vi "Single Point CW.vi"() -> ()   [LabVIEW 2020]
uses:
  Labview Library/Libraries/Basic Experiment/CW Results.ctl
  Labview Library/Libraries/Basic Experiment/CW Fit Frequency.ctl
  <vilib>/Math Plots/2D Math Plots/2D Error Bar/2D Error Bar XCtrl/2D Error Bar.xctl
  <vilib>/Math Plots/2D Math Plots/2D Error Bar/2D Error Bar Datatype/2D Error Bar Datatype.lvclass
  Labview Library/Libraries/Basic Experiment/CW settings.ctl
  Labview Library/Libraries/Basic Experiment/AutoTrace Setting For Exp.ctl
  Labview Library/Libraries/HW_LMMR_ASG8100/LMMR ASG/ASG Instructions XControl.xctl
  <vilib>/Analysis/baseanly.llb/Mean (DBL).vi
  <vilib>/Math Plots/2D Math Plots/2D Error Bar/2D Error Bar Datatype/Public/Plot Helper (Percentage).vi
  Labview Library/Libraries/Basic Experiment/Basic Experiment.lvlib
  Labview Library/Libraries/UT_Utilities/Utilities.lvlib
  Labview Library/Libraries/HW_LMMR_ASG8100/LMMR ASG/ASG 8100 Module.lvlib
  Labview Library/Libraries/HW_NI_CTR/NI DAQ Counter/NI DAQ Counter.lvlib
  <vilib>/Analysis/NI_AALBase.lvlib
  Labview Library/Libraries/HW_Rigol_DSG/Rigol Signal Generator Module/Rigol Signal Generator Module.lvlib
panel:
  in  "?":enum32{"CW Sequence", "CW Spectrum CY", "Check"}(tab)=enum."CW Spectrum CY"
  in  "CW seq":T3(xcontrol)=[{"Flags"=[TRUE, FALSE, FALSE, FALSE, FALSE, FALSE, FALSE, FALSE, FALSE, FALSE, FALSE, FALSE, FALSE, FALSE], "Comments"="", "Time"=2e-06, "Loop Config"={"Loop Code"=enum."Continued", "Number of Loop"=0, "End of Loop"=nan, "Loop Info"=""}}, {"Flags"=[TRUE, FALSE, TRUE, FALSE, FALSE, FALSE, FALSE, FALSE, FALSE, FALSE, FALSE, FALSE, FALSE, FALSE], "Comments"="", "Time"=5e-08, "Loop Config"={"Loop Code"=enum."Continued", "Number of Loop"=0, "End of Loop"=nan, "Loop Info"=""}}, {"Flags"=[TRUE, TRUE, FALSE, FALSE, FALSE, FALSE, FALSE, FALSE, FALSE, FALSE, FALSE, FALSE, FALSE, FALSE], "Comments"="", "Time"=5e-05, "Loop Config"={"Loop Code"=enum."Continued", "Number of Loop"=0, "End of Loop"=nan, "Loop Info"=""}}, {"Flags"=[TRUE, FALSE, TRUE, FALSE, FALSE, FALSE, FALSE, FALSE, FALSE, FALSE, FALSE, FALSE, FALSE, FALSE], "Comments"="", "Time"=5e-08, "Loop Config"={"Loop Code"=enum."Continued", "Number of Loop"=0, "End of Loop"=nan, "Loop Info"=""}}, {"Flags"=[TRUE, FALSE, FALSE, FALSE, FALSE, FALSE, FALSE, FALSE, TRUE, FALSE, FALSE, FALSE, FALSE, FALSE], "Comments"="", "Time"=2e-06, "Loop Config"={"Loop Code"=enum."Continued", "Number of Loop"=0, "End of Loop"=nan, "Loop Info"=""}}, {"Flags"=[TRUE, FALSE, TRUE, FALSE, FALSE, FALSE, FALSE, FALSE, FALSE, FALSE, FALSE, FALSE, FALSE, FALSE], "Comments"="", "Time"=5e-08, "Loop Config"={"Loop Code"=enum."Continued", "Number of Loop"=0, "End of Loop"=nan, "Loop Info"=""}}, {"Flags"=[TRUE, FALSE, FALSE, FALSE, FALSE, FALSE, FALSE, FALSE, FALSE, FALSE, FALSE, FALSE, FALSE, FALSE], "Comments"="", "Time"=5e-05, "Loop Config"={"Loop Code"=enum."Continued", "Number of Loop"=0, "End of Loop"=nan, "Loop Info"=""}}, {"Flags"=[TRUE, FALSE, TRUE, FALSE, FALSE, FALSE, FALSE, FALSE, FALSE, FALSE, FALSE, FALSE, FALSE, FALSE], "Comments"="", "Time"=5e-08, "Loop Config"={"Loop Code"=enum."Continued", "Number of Loop"=0, "End of Loop"=nan, "Loop Info"=""}}, {"Flags"=[TRUE, FALSE, FALSE, FALSE, FALSE, FALSE, FALSE, FALSE, FALSE, FALSE, FALSE, FALSE, FALSE, FALSE], "Comments"="", "Time"=2e-06, "Loop Config"={"Loop Code"=enum."Continued", "Number of Loop"=0, "End of Loop"=nan, "Loop Info"=""}}]
  out "Is NV?":bool
  out "Signal and Ref":cluster{"Numeric":dbl, "Numeric":dbl}(graph)={"Numeric"=21362.166666666664, "Numeric"=24241.083333333332}
  in  "Settings":T4={"Num Pts"=20, "Start freq"=1374.6, "Stop freq"=1374.6, " dBm"=-7.0, "Ratio \nThre(abs)"=0.03, "AutoTrace Before Exp"=FALSE, "RepoSave"=FALSE, "Peak Num \nLimit "=2, "Loop per Update"=12000, "UpdateTime"=20} {"UpdateTime" format="%.0p"; "Loop per Update" format="%#_6p"}
  in  "AutoTrace Settings":T5={"Ratio"=0.5, "Threshold"=12673.708333333332, "Trace Times"=58, "Max Times"=100, "AutoTrace Status"=enum."Normal"}
  out "Total Time (min)":ext=8.9208000000000003786 format="%#.5p"
  out "Readout Result":refnum<class "2D Plot Datatype.lvclass">[](xcontrol) caption="2D Error Bar"
  out "CW Result":T6={"Fit Frequency"={"Fre2"={"Amplitude"=nan, "Position"=nan, "Width"=nan}, "Fre1"={"Amplitude"=nan, "Position"=nan, "Width"=nan}, "Fre3"={"Amplitude"=nan, "Position"=nan, "Width"=nan}, "Background"=nan}, "Pro"=[-0.12635567482468857, -0.1267749409899792, -0.12303982094908628, -0.12479221956785369, -0.12201167231342569, -0.12661611896327096, -0.12133042096022884, -0.11895379638798553, -0.12207791874792728, -0.11872317522087106], "Error Bar"=[0.0023197288862702743, 0.0023236987167363893, 0.002342167656034516, 0.0023395461288415573, 0.0023484887471034014, 0.002342726319419302, 0.0023787761645139233, 0.0024016586189280643, 0.002379318052297366, 0.002387271904965039], "Raw Data Path"=path "G:/Raw Data/RawTdms/Y2024M03D11/ Single Point CW Y2024M03D11_11_31_34 SN23_07_27_ 326.tdms", "Image Path"=path "G:/Raw Data/RawImage/Y2024M03D11/ Single Point CW Y2024M03D11_11_31_34 SN23_07_27_ 326.png"}
  out "Fre sequence":dbl[](array[numeric])=[1374.6, 1374.6, 1374.6, 1374.6, 1374.6, 1374.6, 1374.6, 1374.6, 1374.6, 1374.6, 1374.6, 1374.6, 1374.6, 1374.6, 1374.6, 1374.6, 1374.6, 1374.6, 1374.6, 1374.6, 1374.6]
  out "Pro Array":dbl[](array[numeric])=[-0.12635567482468857, -0.1267749409899792, -0.12303982094908628, -0.12479221956785369, -0.12201167231342569, -0.12661611896327096, -0.12133042096022884, -0.11895379638798553, -0.12207791874792728, -0.11872317522087106]
  in  "error in (no error)":errorcluster
  out "error out":errorcluster
  # "CW Settings"
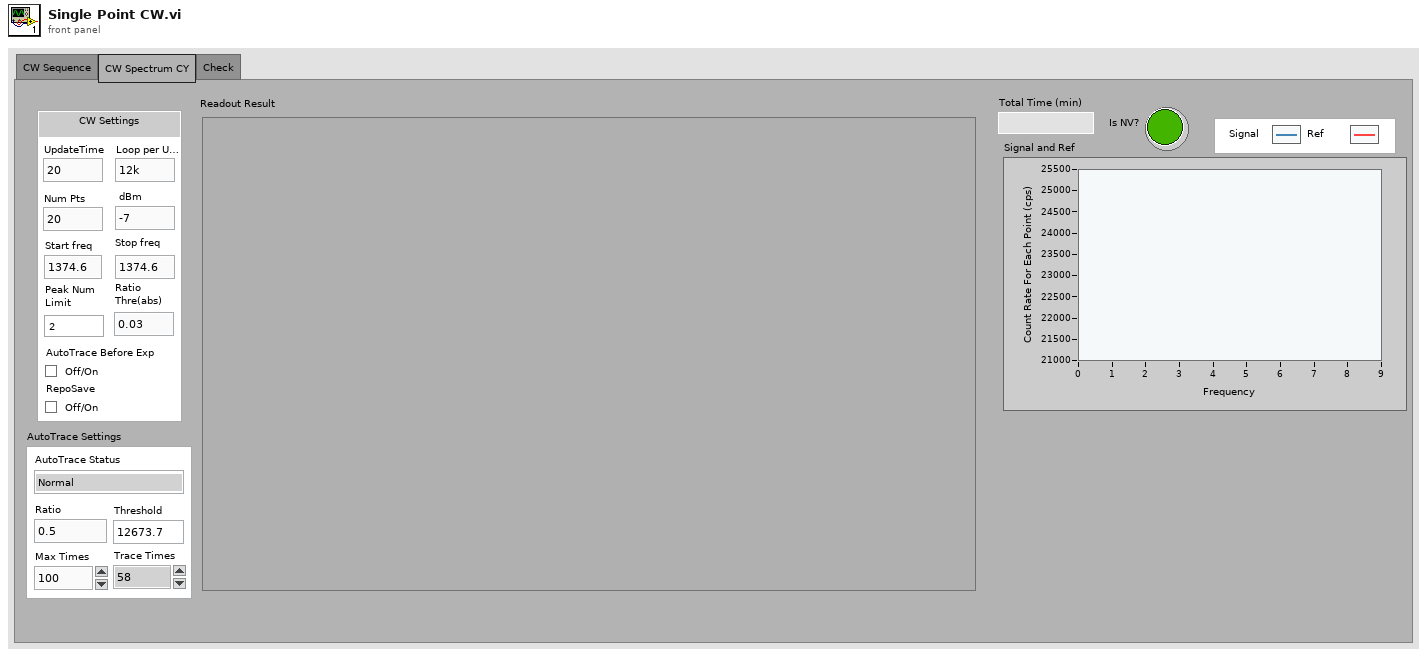
[diagram p1: front panel]
types:
  T1 = typedef "Loop XControl.xctl/Loop Config.ctl" = cluster{"Loop Code":T2, "Number of Loop":i32, "End of Loop":dbl, "Loop Info":string}
  T2 = typedef "Loop XControl.xctl/Loop Code.ctl" = enum16{"Continued", "Loop", "End Loop"}
  T3 = cluster{"Flags":bool[], "Comments":string, "Time":dbl, "Loop Config":T1}[]
  T4 = typedef "Basic Experiment.lvlib/CW settings.ctl" = cluster{"Num Pts":i32, "Start freq":dbl, "Stop freq":dbl, " dBm":dbl, "Ratio \nThre(abs)":dbl, "AutoTrace Before Exp":bool, "RepoSave":bool, "Peak Num \nLimit ":i32, "Loop per Update":u32, "UpdateTime":i32}
  T5 = typedef "Basic Experiment.lvlib/AutoTrace Setting For Exp.ctl" = cluster{"Ratio":dbl, "Threshold":dbl, "Trace Times":i32, "Max Times":i32, "AutoTrace Status":enum16{"Normal", "AutoTrace  Last Loop", "Unintialized"}}
  T6 = typedef "Basic Experiment.lvlib/CW Results.ctl" = cluster{"Fit Frequency":T7, "Pro":dbl[], "Error Bar":dbl[], "Raw Data Path":path, "Image Path":path}
  T7 = typedef "Basic Experiment.lvlib/CW Fit Frequency.ctl" = cluster{"Fre2":cluster{"Amplitude":dbl, "Position":dbl, "Width":dbl}, "Fre1":cluster{"Amplitude":dbl, "Position":dbl, "Width":dbl}, "Fre3":cluster{"Amplitude":dbl, "Position":dbl, "Width":dbl}, "Background":dbl}
  T8 = enum16{"Normal", "AutoTrace  Last Loop", "Unintialized"}
  T9 = enum16{"open", "open or create", "create or replace", "create", "open (read-only)"}
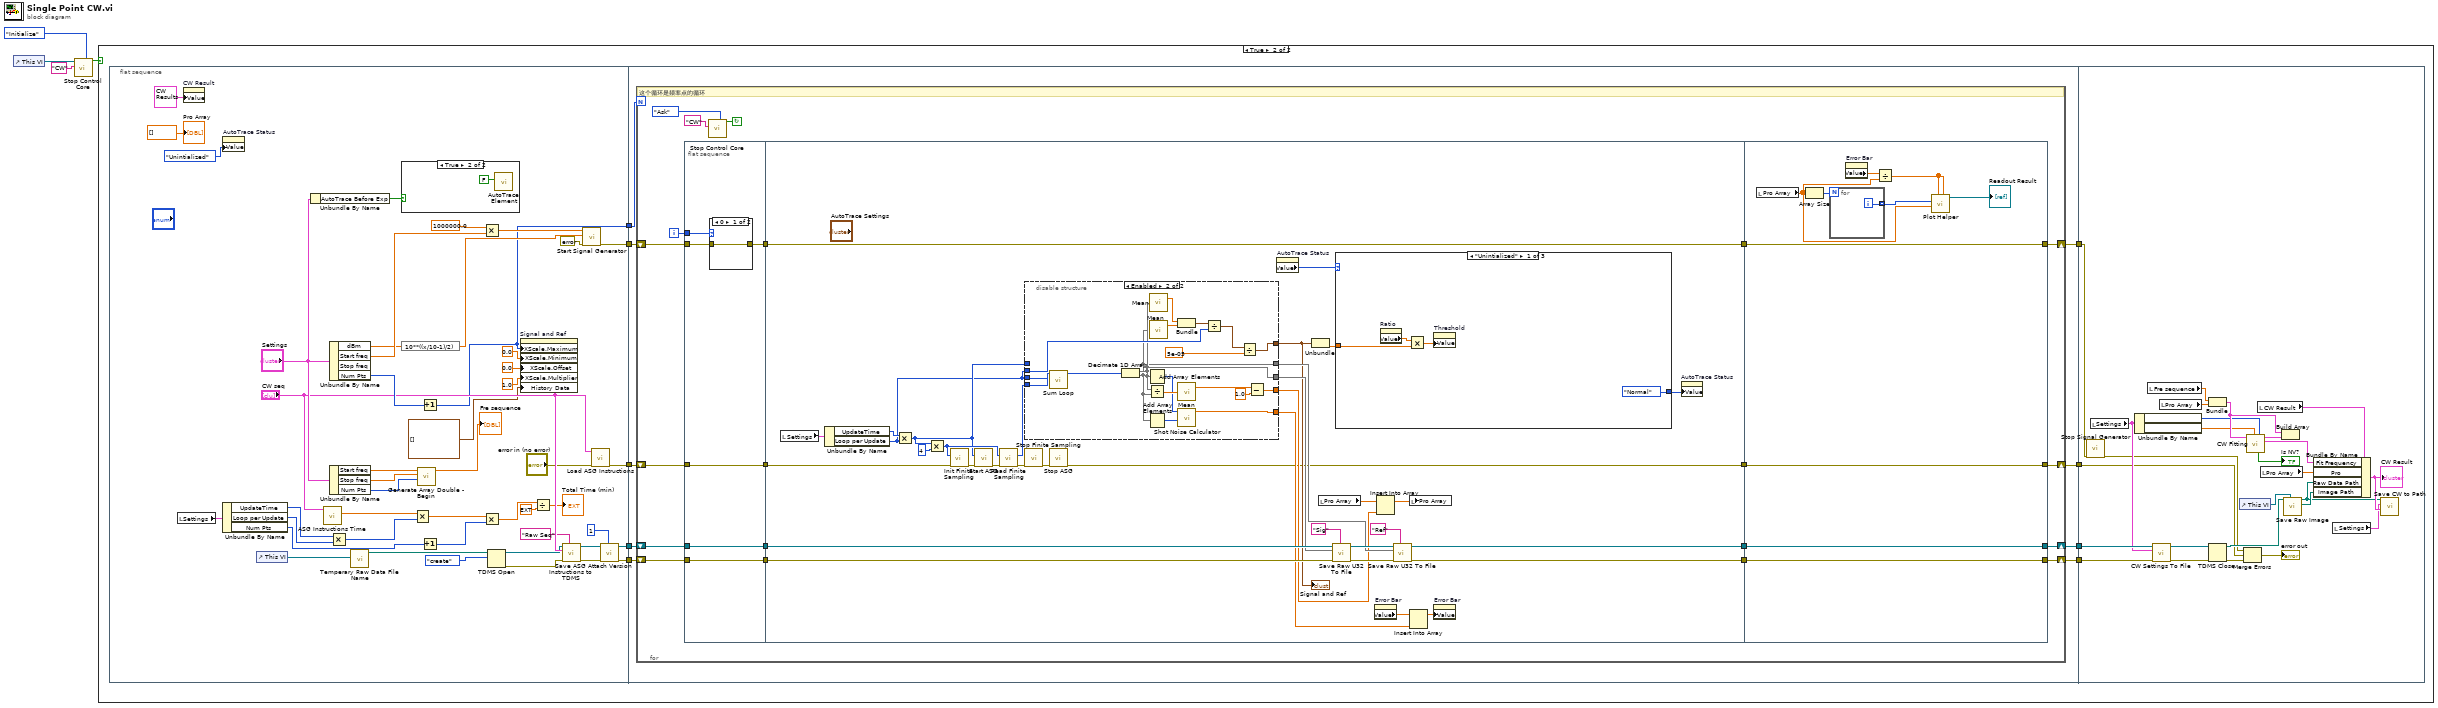
[diagram p0: block diagram]
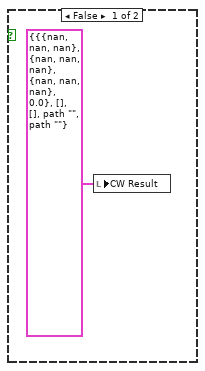
[diagram p2: hidden frame]
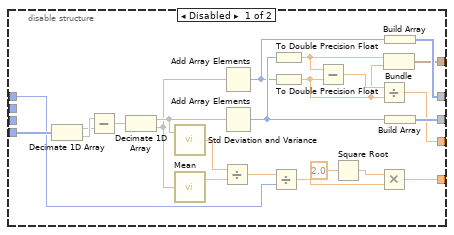
[diagram p5: hidden frame]
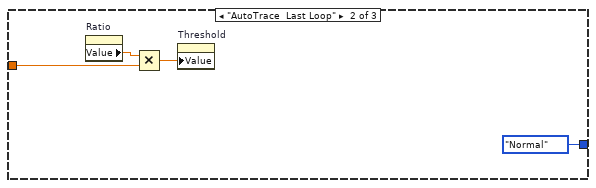
[diagram p6: hidden frame]
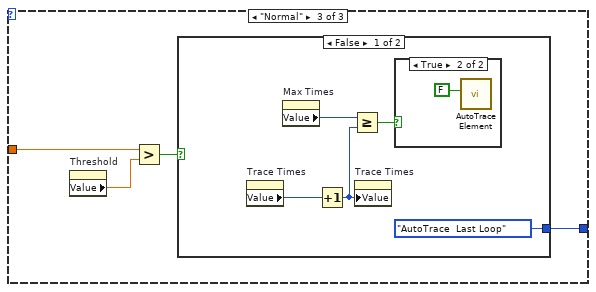
[diagram p7: hidden frame]
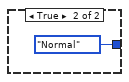
[diagram p9: hidden frame]
diagram:
  n1 = control-ref of="This VI"() -> (w3:refnum<vi>)
  n2 = call "Stop Control Core.vi"("Mode"=enum16{"Ask", "Initialize"}."Initialize", "Program Name"="CW", "VI Ref"=w3) -> ("Continue Sign(Continue:True)"=w1:bool)  [unwired: 8 in]
  n3 = case shown="True" w1 {
    frame False {
      n4 = local write "CW Result"(T6 {"Fit Frequency"={"Fre2"={"Amplitude"=nan, "Position"=nan, "Width"=nan}, "Fre1"={"Amplitude"=nan, "Position"=nan, "Width"=nan}, "Fre3"={"Amplitude"=nan, "Position"=nan, "Width"=nan}, "Background"=0.0}, "Pro"=[], "Error Bar"=[], "Raw Data Path"=path "", "Image Path"=path ""} ("CW Result")) -> ()
    }
    frame True {
      n5 = flat-sequence {
        tunnel: [w26] -> w11
        tunnel: [w16] -> w10
        tunnel: [w30] -> w9
        tunnel: [w29] -> w8
        tunnel: [w28] -> w7
        tunnel: [w71] -> w14
        tunnel: [w70] -> w13
        tunnel: [w69] -> w12
        tunnel: w11 -> [w68]
        tunnel: w10 -> [w67]
        tunnel: w9 -> [w66]
        tunnel: w8 -> [w65]
        tunnel: w7 -> [w64]
        tunnel: [w63] -> w6
        tunnel: w14 -> [w228]
        tunnel: w13 -> [w227]
        tunnel: w12 -> [w210]
        tunnel: w6 -> [w208]
        frame #0 {
          n6 = local read "Settings"() -> (w39:T4)
          n7 = property on="CW Result" class="Clust (strict)"("Value"=T6 {"Fit Frequency"={"Fre2"={"Amplitude"=nan, "Position"=nan, "Width"=nan}, "Fre1"={"Amplitude"=nan, "Position"=nan, "Width"=nan}, "Fre3"={"Amplitude"=nan, "Position"=nan, "Width"=nan}, "Background"=0.0}, "Pro"=[], "Error Bar"=[], "Raw Data Path"=path "", "Image Path"=path ""} ("CW Result")) -> ()  [unwired: 2 in, 2 out]
          n8 = property on="AutoTrace Status" class="Enum (strict)"("Value"=T8."Unintialized") -> ()  [unwired: 2 in, 2 out]
          n9 = Unbundle By Name(w39) -> ("UpdateTime"=w47:i32, "Loop per Update"=w48:u32, "Num Pts"=w42:i32)
          n10 = control-ref of="This VI"() -> (w34:refnum<vi>)
          n11 = Unbundle By Name("Settings") -> ("AutoTrace Before Exp"=w57:bool)
          n12 = call "ASG Instructions Time.vi"("ASG Instr. A"="CW seq") -> ("Total Time (s)"=w41:ext)  [unwired: 10 in]
          n13 = Unbundle By Name("Settings") -> ("dBm"=w51:dbl, "Start freq"=w53:dbl, "Num Pts"=w52:i32)  [unwired: 1 out]
          n14 = Unbundle By Name("Settings") -> ("Start freq"=w61:dbl, "Stop freq"=w60:dbl, "Num Pts"=w55:i32)
          n15 = Multiply(x=w47, y=w48) -> (x*y=w49:u32)
          n16 = call "Temperary Raw Data File Name.vi"("VI ref"=w34) -> ("Raw data Path"=w35:path)  [unwired: 10 in]
          n17 = case shown="True" w57 {
            frame False {
            }
            frame True {
              n18 = call "AutoTrace Element.vi"("Need Correct Count?(T)"=FALSE) -> ()  [unwired: 9 in, 2 out]
            }
          }
          n19 = expression code="10**((x/10-1)/2)"(w51) -> (w27:dbl)
          n20 = Multiply(x=w41, y=w49) -> (x*y=w43:ext)
          n21 = call "Generate Array Double - Begin.vi"("num of step"=w55, "end"=w60, "begin"=w61) -> ("output array"=→"Fre sequence":dbl[])  [unwired: 5 in, 3 out]
          n22 = Increment(x=w52) -> (x+1=w16:i32)
          n23 = Increment(x=w42) -> (x+1=w44:i32)
          n24 = Multiply(x=1000000.0, y=w53) -> (x*y=w25:dbl)
          n25 = Multiply(x=w43, y=w44) -> (x*y=w22:ext)
          n26 = TDMS Open(10:T9."create" ("operation (0:open)"), 11:w35) -> (0:w37:errorcluster, 3:w36:refnum<k34>)  [unwired: 5 in]
          n27 = property on="Signal and Ref" class="WFChart (strict)"("XScale.Maximum"=w16, "XScale.Minimum"=0.0 ("X Scale.Range:Minimum"), "XScale.Offset"=0.0 ("X Scale.Offset and Multiplier:Offset"), "XScale.Multiplier"=1.0 ("X Scale.Offset and Multiplier:Multiplier"), "History Data"=cluster{"Signal":dbl, "Ref":dbl}[] []) -> ()  [unwired: 2 in, 2 out]
          n28 = Divide(x=w22, y=ext 60.0) -> (x/y=→"Total Time (min)":ext)
          n29 = call "Save ASG Instructions to TDMS.vi"("Name"="Raw Seq", "error in (no error)"=w37, "ASG Instructions"="CW seq", "tdms file"=w36) -> ("error out"=w46:errorcluster, "tdms file out"=w45:refnum<k34>)  [unwired: 6 in]
          n30 = call "Start Signal Generator.vi"("error in"=errorcluster {"status"=FALSE, "code"=0, "source"=""}, "Amplitude (V)"=w27, "Frequency (Hz)"=w25) -> ("error out"=w26:errorcluster)  [unwired: 7 in, 1 out]
          n31 = call "Load ASG Instructions.vi"("error in (no error)"="error in (no error)", "ASG Instructions"="CW seq") -> ("error out"=w30:errorcluster)  [unwired: 9 in]
          n32 = call "Attach Version.vi"("Version"=u32 1, "error in (no error)"=w46, "Refnum in"=w45) -> ("error out"=w29:errorcluster, "Refnum out"=w28:refnum<k34>)  [unwired: 5 in, 2 out]
          "Pro Array" <- dbl[] [] ("Pro Array")
        }
        frame #1 {
          n33 = for {
            N: w67 -> [_]
            shift-right: [w87] -> w70
            shift-left: w65 -> [w90]
            shift-right: [w88] -> w71
            shift-left: w64 -> [w86]
            shift-right: [w76] -> w69
            shift-left: w68 -> [w79]
            shift-right: [w72] -> w63
            shift-left: w66 -> [w74]
            i -> [w75]
            stop <- w83 continue-if-true
            # "这个循环是频率点的循环"
            n34 = flat-sequence {
              tunnel: w86 -> [w97]
              tunnel: [w97] -> w91
              tunnel: w90 -> [w96]
              tunnel: [w96] -> w89
              tunnel: [w92] -> w80
              tunnel: w79 -> [w95]
              tunnel: [w94] -> w77
              tunnel: w75 -> [w93]
              tunnel: w74 -> [w92]
              tunnel: w89 -> [w122]
              tunnel: w91 -> [w123]
              tunnel: [w118] -> w82
              tunnel: [w120] -> w81
              tunnel: w80 -> [w106]
              tunnel: [w102] -> w78
              tunnel: w77 -> [w102]
              tunnel: [w101] -> w73
              tunnel: [w203] -> w87
              tunnel: [w204] -> w88
              tunnel: w82 -> [w204]
              tunnel: w81 -> [w203]
              tunnel: [w199] -> w76
              tunnel: w78 -> [w199]
              tunnel: w73 -> [w198]
              tunnel: [w198] -> w72
              frame #0 {
                n35 = case shown="0" w93 {
                  tunnel: w95 -> [w98 w99]
                  tunnel: [w98 w99] -> w94
                  frame 0 {
                  }
                  frame 1, Default {
                  }
                }
              }
              frame #1 {
                n36 = local read "Settings"() -> (w115:T4)
                n37 = Unbundle By Name(w115) -> ("UpdateTime"=w107:i32, "Loop per Update"=w105:u32)
                n38 = Multiply(x=w107, y=w105) -> (x*y=w108:u32)
                n39 = Multiply(x=w108, y=4) -> (x*y=w128:u32)
                n40 = call "Init Finite Sampling.vi"("error in"=w106, "Num of Sample"=w128) -> ("error out"=w125:errorcluster)  [unwired: 9 in]
                n41 = call "Start ASG.vi"("error in (no error)"=w125, "Loop Number"=w108) -> ("error out"=w124:errorcluster)  [unwired: 8 in, 1 out]
                n42 = call "Read Finite Sampling.vi"("error in"=w124, "Samples to Read"=w128) -> ("error out"=w129:errorcluster, "Sample Array"=w133:u32[])  [unwired: 7 in, 1 out]
                n43 = disable-structure shown="Enabled" {
                  disable-tunnel: w133 -> [w154 w175]
                  disable-tunnel: w105 -> [_ w174]
                  disable-tunnel: [w149 w161] -> w112
                  disable-tunnel: [w148 w160] -> w111
                  disable-tunnel: [w145 w169] -> w110
                  disable-tunnel: w108 -> [w137 _]
                  disable-tunnel: [w135 w157] -> w109
                  disable-tunnel: [w134 w162] -> w104
                  disable-tunnel: w105 -> [_ w165]
                  frame Disabled {
                    n44 = Decimate 1D Array(w154) -> (w155:u32[], w156:u32[])
                    n45 = Subtract(x=w156, y=w155) -> (x-y=w153:u32[])
                    n46 = Decimate 1D Array(w153) -> (w150:u32[], w147:u32[])
                    n47 = call <vilib>:"Std Deviation and Variance.vi"("X"=w150) -> ("standard deviation"=w139:dbl)  [unwired: 1 in, 2 out]
                    n48 = call-poly <vilib>:"Mean.vi"("X"=w147) -> ("mean"=w136:dbl)  [unwired: 1 out]
                    n49 = Divide(x=w139, y=w136) -> (x/y=w140:dbl)
                    n50 = Add Array Elements(numeric array=w147) -> (sum=w151:u32)
                    n51 = Add Array Elements(numeric array=w150) -> (sum=w152:u32)
                    n52 = Divide(x=w140, y=w137) -> (x/y=w142:dbl)
                    n53 = To Double Precision Float(number=w152) -> (double precision float=w143:dbl)
                    n54 = To Double Precision Float(number=w151) -> (double precision float=w144:dbl)
                    n55 = Subtract(x=w143, y=w144) -> (x-y=w146:dbl)
                    n56 = Square Root(x=2.0) -> (sqrt(x)=w141:dbl)
                    n57 = Divide(x=w146, y=w144) -> (x/y=w145:dbl)
                    n58 = Multiply(x=w141, y=w142) -> (x*y=w135:dbl)
                    n59 = Bundle(w143, w144) -> (w134:cluster{dbl, dbl})  [unwired: 1 in]
                    n60 = Build Array(w151) -> (w148:u32[])
                    n61 = Build Array(w152) -> (w149:u32[])
                  }
                  frame Enabled {
                    n62 = call "Sum Loop.vi"("Loop per Update"=w174, "Raw Data Array"=w175) -> ("Data after sum"=w173:u32[])  [unwired: 9 in]
                    n63 = Decimate 1D Array(w173) -> (w161:u32[], w160:u32[])
                    n64 = Add Array Elements(numeric array=w161) -> (sum=w159:u32)
                    n65 = Divide(x=w161, y=w160) -> (x/y=w172:dbl[])
                    n66 = Add Array Elements(numeric array=w160) -> (sum=w158:u32)
                    n67 = call-poly <vilib>:"Mean.vi"("X"=w161) -> ("mean"=w168:dbl)  [unwired: 1 out]
                    n68 = call-poly <vilib>:"Mean.vi"("X"=w160) -> ("mean"=w167:dbl)  [unwired: 1 out]
                    n69 = Bundle("mean"=w168, "mean"=w167) -> (w166:cluster{"mean":dbl, "mean":dbl})  [unwired: 1 in]
                    n70 = call-poly <vilib>:"Mean.vi"("X"=w172) -> ("mean"=w171:dbl)  [unwired: 1 out]
                    n71 = call "Shot Noise Calculator.vi"("Toral Ref Count"=w158, "Total Sig Count"=w159) -> ("Error Given By ShotNoise"=w157:dbl)  [unwired: 9 in]
                    n72 = Divide(x=w166, y=w165) -> (x/y=w164:cluster{"mean":dbl, "mean":dbl})
                    n73 = Divide(x=w164, y=5e-05) -> (x/y=w162:cluster{"mean":dbl, "mean":dbl})
                    n74 = Subtract(x=w171, y=1.0) -> (x-y=w169:dbl)
                  }
                }
                "Signal and Ref" <- w104
                n75 = call "Stop Finite Sampling.vi"("error in"=w129) -> ("error out"=w126:errorcluster)  [unwired: 10 in]
                n76 = call "Stop ASG.vi"("error in (no error)"=w126) -> ("error out"=w101:errorcluster)  [unwired: 9 in, 1 out]
                n77 = property on="AutoTrace Status" class="Enum (strict)"() -> ("Value"=w100:T8)  [unwired: 2 in, 2 out]
                n78 = Unbundle(w104) -> ("mean"=w103:dbl)  [unwired: 1 out]
                n79 = local read "Pro Array"() -> (w132:dbl[])
                n80 = call "Save Raw U32 To File.vi"("Suffix"="Sig" ("PS"), "error in"=w122, "Sample Array"=w112, "Refnum in"=w123) -> ("error out"=w121:errorcluster, "tdms file out"=w119:refnum<k34>)  [unwired: 4 in, 2 out]
                n81 = case shown="\"Unintialized\"" w100 {
                  tunnel: [T8."Normal" ("Enum") T8."Normal" ("Enum") w187] -> w130
                  tunnel: w103 -> [w177 w181 w186]
                  frame "Unintialized" {
                    n82 = property on="Ratio" class="DigNum (strict)"() -> ("Value"=w176:dbl)  [unwired: 2 in, 2 out]
                    n83 = Multiply(x=w176, y=w177) -> (x*y=w178:dbl)
                    n84 = property on="Threshold" class="DigNum (strict)"("Value"=w178) -> ()  [unwired: 2 in, 2 out]
                  }
                  frame "AutoTrace  Last Loop" {
                    n85 = property on="Ratio" class="DigNum (strict)"() -> ("Value"=w183:dbl)  [unwired: 2 in, 2 out]
                    n86 = Multiply(x=w183, y=w181) -> (x*y=w182:dbl)
                    n87 = property on="Threshold" class="DigNum (strict)"("Value"=w182) -> ()  [unwired: 2 in, 2 out]
                  }
                  frame "Normal" {
                    n88 = property on="Threshold" class="DigNum (strict)"() -> ("Value"=w184:dbl)  [unwired: 2 in, 2 out]
                    n89 = Greater?(x=w186, y=w184) -> (0:w185:bool)
                    n90 = case shown="False" w185 {
                      tunnel: [T8."AutoTrace  Last Loop" ("Enum") T8."Normal" ("Enum")] -> w187
                      frame False {
                        n91 = property on="Trace Times" class="DigNum (strict)"() -> ("Value"=w188:i32)  [unwired: 2 in, 2 out]
                        n92 = property on="Max Times" class="DigNum (strict)"() -> ("Value"=w190:i32)  [unwired: 2 in, 2 out]
                        n93 = Increment(x=w188) -> (x+1=w191:i32)
                        n94 = Greater Or Equal?(x=w190, y=w191) -> (x >= y?=w189:bool)
                        n95 = property on="Trace Times" class="DigNum (strict)"("Value"=w191) -> ()  [unwired: 2 in, 2 out]
                        n96 = case shown="True" w189 {
                          frame False {
                          }
                          frame True {
                            n97 = call "AutoTrace Element.vi"("Need Correct Count?(T)"=FALSE) -> ()  [unwired: 9 in, 2 out]
                          }
                        }
                      }
                      frame True {
                      }
                    }
                  }
                }
                n98 = property on="Error Bar" class="Arr (strict)"() -> ("Value"=w117:dbl[])  [unwired: 2 in, 2 out]
                n99 = Insert Into Array(array=w132, new element=w110) -> (w131:dbl[])  [unwired: 1 in]
                n100 = call "Save Raw U32 To File.vi"("Suffix"="Ref" ("PS"), "error in"=w121, "Sample Array"=w111, "Refnum in"=w119) -> ("error out"=w120:errorcluster, "tdms file out"=w118:refnum<k34>)  [unwired: 4 in, 2 out]
                n101 = local write "Pro Array"(w131) -> ()
                n102 = Insert Into Array(array=w117, new element=w109) -> (w116:dbl[])  [unwired: 1 in]
                n103 = property on="Error Bar" class="Arr (strict)"("Value"=w116) -> ()  [unwired: 2 in, 2 out]
                n104 = property on="AutoTrace Status" class="Enum (strict)"("Value"=w130) -> ()  [unwired: 2 in, 2 out]
              }
              frame #2 {
                n105 = local read "Pro Array"() -> (w197:dbl[])
                n106 = Array Size(array=w197) -> (size(s)=w196:i32)
                n107 = for {
                  N: w196 -> [_]
                  tunnel: [w205] -> w195 mode=indexing
                  i -> [w205]
                }
                n108 = property on="Error Bar" class="Arr (strict)"() -> ("Value"=w200:dbl[])  [unwired: 2 in, 2 out]
                n109 = Divide(x=w200, y=w197) -> (x/y=w202:dbl[])
                n110 = call-poly <vilib>:"Plot Helper.vi"("error b percentage"=w202, "error a percentage"=w202, "y vector"=w197, "x vector"=w195) -> ("2D Plot Class Obj Array out"=→"Readout Result":refnum<class "2D Plot Datatype.lvclass">[])  [unwired: 2 in, 5 out]
              }
            }
            n111 = call "Stop Control Core.vi"("Mode"=enum16{"Ask", "Initialize"}."Ask", "Program Name"="CW") -> ("Continue Sign(Continue:True)"=w83:bool)  [unwired: 9 in]
          }
        }
        frame #2 {
          n112 = call "Stop Signal Generator.vi"("error in"=w210) -> ("error out"=w207:errorcluster)  [unwired: 9 in, 1 out]
          n113 = local read "Settings"() -> (w216:T4)
          n114 = Unbundle By Name(w216) -> ("Peak Num \nLimit"=w214:i32, "Ratio \nThre(abs)"=w215:dbl)
          n115 = local read "Fre sequence"() -> (w231:dbl[])
          n116 = call "CW Settings To File.vi"("error in (no error)"=w227, "CW settings"=w216, "tdms file"=w228) -> ("error out"=w225:errorcluster, "tdms file out"=w226:refnum<k34>)  [unwired: 7 in]
          n117 = local read "Pro Array"() -> (w230:dbl[])
          n118 = Bundle("Fre sequence"=w231, "Pro Array"=w230) -> (w229:cluster{"Fre sequence":dbl[], "Pro Array":dbl[]})  [unwired: 1 in]
          n119 = TDMS Close(8:w225, 11:w226) -> (0:w206:errorcluster, 3:w223:path)
          n120 = control-ref of="This VI"() -> (w224:refnum<vi>)
          n121 = Merge Errors(w207, w208, w206) -> (→"error out":errorcluster)
          n122 = call "CW Fitting.vi"("Peak Num Limit"=w214, "Ratio Thre(abs)"=w215, "Origin Data"=w229) -> ("Fit Frequency"=w211:T7, "Fit Curve"=w213:cluster{"x":dbl[], "y":dbl[]}, "Is NV?"=→"Is NV?":bool)  [unwired: 5 in, 1 out]
          n123 = local read "CW Result"() -> (w217:T6)
          n124 = local read "Pro Array"() -> (w222:dbl[])
          n125 = Build Array(w229, w213) -> ()  [unwired: 1 out]
          n126 = call "Save Raw Image.vi"("reference"=w224, "Raw TDMS Path"=w223) -> ("Image Path"=w221:path, "Raw TDMS Path Out"=w218:path)  [unwired: 7 in, 1 out]
          n127 = Bundle By Name(cluster=w217, "Fit Frequency"=w211, "Pro"=w222, "Raw Data Path"=w218, "Image Path"=w221) -> (w220:T6)
          "CW Result" <- w220
          n128 = local read "Settings"() -> (w219:T4)
          n129 = call "Save CW to Path.vi"("CW Result"=w220, "setting section"=w219, "file path"=w218) -> ()  [unwired: 5 in, 4 out]
        }
      }
    }
  }
